vi "Load_USB_DAQ_Config_File.vi"(1 "App Path":path) -> (0 "USB DAQ Vsup":dbl min=0.0 max=5.0, 2 "USB DAQ Address":i32, 3 "DAC Mode":i32, 4 "ADS Mode":i32, 5 "USB DAQ Vref":dbl min=0.0 max=5.0)   [LabVIEW 2011]
doc: "1. This VI will read the USB-DAQ configure file \"USB_DAQ.ini\". This file keeps key variables required to use the USB-DAQ (e.g. USB address). \n2. If the file does not exist, the VI will create the file and folder. The folder is \"Config_Files\".\n3. When the program is closed, a different VI (\"save_usb_config_file.vi\") will save any changes made to the USB-DAQ configuration."
uses:
  INA231/Global 1.vi
  <vilib>/Utility/config.llb/Read Key (Double).vi
  <vilib>/Utility/config.llb/Read Key (I32).vi
  <vilib>/Utility/config.llb/NI_LVConfig.lvlib
panel:
  # "Outputs"
  # "Inputs"
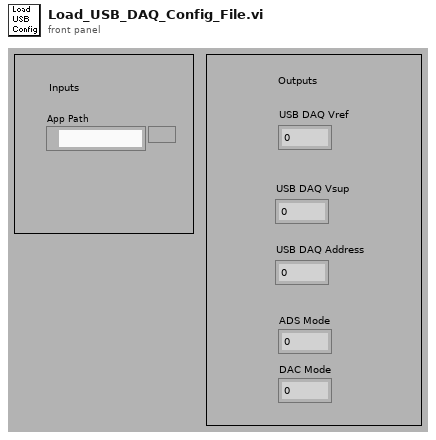
[diagram p1: front panel]
types:
  T1 = typedef "NI_LVConfig.lvlib/Config Data RefNum.ctl" = refnum<k1>
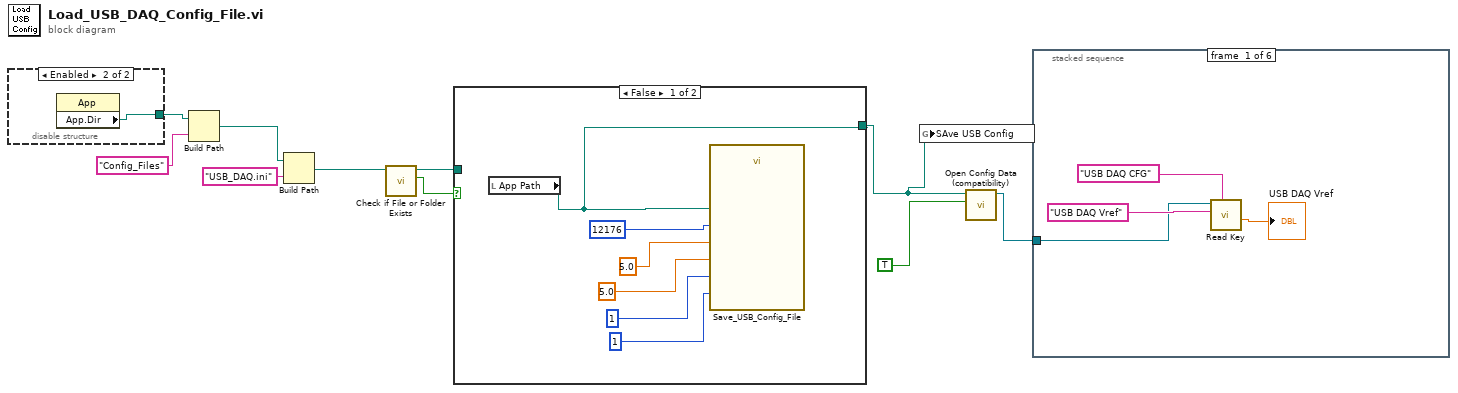
[diagram p0: block diagram]
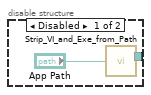
[diagram p2: hidden frame]
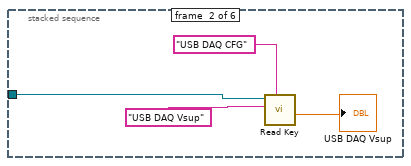
[diagram p4: hidden frame]
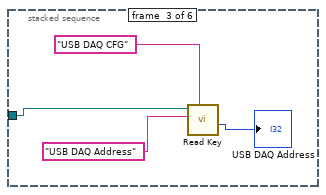
[diagram p5: hidden frame]
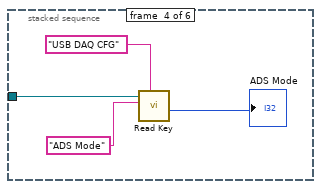
[diagram p6: hidden frame]
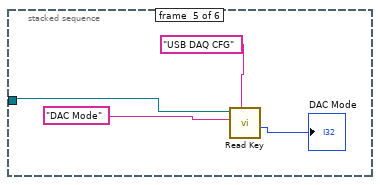
[diagram p7: hidden frame]
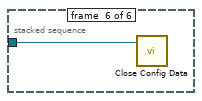
[diagram p8: hidden frame]
diagram:
  n1 = disable-structure shown="Enabled" {
    disable-tunnel: [w12 w13] -> w2
    frame Disabled {
      n2 = call "Strip_VI_and_Exe_from_Path.vi"("App Path"="App Path") -> ("App Path out"=w12:path)
    }
    frame Enabled {
      n3 = property class="App"() -> ("App.Dir"=w13:path)  [unwired: 2 in, 2 out]
    }
  }
  n4 = Build Path(base path=w2, name or relative path="Config_Files") -> (appended path=w8:path)
  n5 = Build Path(base path=w8, name or relative path="USB_DAQ.ini") -> (appended path=w7:path)
  n6 = call <vilib>:"Check if File or Folder Exists.vi"("path"=w7) -> ("file or folder exists?"=w6:bool, "dup path"=w5:path)  [unwired: 8 in, 1 out]
  n7 = case shown="False" w6 {
    tunnel: w5 -> [_ w20]
    tunnel: [w14 w20] -> w1
    frame False {
      n8 = local read "App Path"() -> (w14:path)
      n9 = call "Save_USB_Config_File.vi"("DAC Mode"=1, "ADS Mode"=1, "USB DAQ Vsup"=5.0, "USB DAQ Vref"=5.0, "USB DAQ Address"=u16 12176, "App Path"=w14) -> ()
    }
    frame True {
    }
  }
  n10 = global write "Global 1.vi" "SAve USB Config"(w1) -> ()
  n11 = call <vilib>:"Open Config Data (compatibility).vi"("create file if necessary (T)"=TRUE ("create file if necessary? (T)"), "configuration file path"=w1) -> ("refnum"=w3:T1)  [unwired: 7 in, 2 out]
  n12 = stacked-sequence {
    tunnel: w3 -> [w23 w28 w32 w36 w40 w41]
    frame #0 {
      n13 = call-poly <vilib>:"Read Key.vi"("section"="USB DAQ CFG", "key"="USB DAQ Vref", "refnum"=w23) -> ("value"=→"USB DAQ Vref":dbl)  [unwired: 5 in, 3 out]
    }
    frame #1 {
      n14 = call-poly <vilib>:"Read Key.vi"("section"="USB DAQ CFG", "key"="USB DAQ Vsup" ("section"), "refnum"=w28) -> ("value"=→"USB DAQ Vsup":dbl)  [unwired: 5 in, 3 out]
    }
    frame #2 {
      n15 = call-poly <vilib>:"Read Key.vi"("section"="USB DAQ CFG", "key"="USB DAQ Address" ("section"), "refnum"=w32) -> ("value"=→"USB DAQ Address":i32)  [unwired: 5 in, 3 out]
    }
    frame #3 {
      n16 = call-poly <vilib>:"Read Key.vi"("section"="USB DAQ CFG", "key"="ADS Mode" ("section"), "refnum"=w36) -> ("value"=→"ADS Mode":i32)  [unwired: 5 in, 3 out]
    }
    frame #4 {
      n17 = call-poly <vilib>:"Read Key.vi"("section"="USB DAQ CFG", "key"="DAC Mode" ("section"), "refnum"=w40) -> ("value"=→"DAC Mode":i32)  [unwired: 5 in, 3 out]
    }
    frame #5 {
      n18 = call <vilib>:"Close Config Data.vi"("refnum"=w41) -> ()  [unwired: 9 in, 2 out]
    }
  }
